vi "Send Connection List.vi"(8 "error in (no error)":errorcluster, 10 "ConnHandlers":refnum<class "Message Enqueuer.lvclass">[](array[class]), 11 "Connection Handler in":refnum<class "Connection Handler.lvclass">) -> (0 "error out":errorcluster, 3 "Connection Handler out":refnum<class "Connection Handler.lvclass">)   [LabVIEW 2017, in "Send Connection List Msg.lvclass"]
uses:
  Connection Handler Messages/Send Connection List Msg/Send Connection List Msg.lvclass
  <vilib>/ActorFramework/Actor/Actor.lvclass
  Connection Handler.lvclass
  Volumes/Data/Users/benji667/Git/BuildFarm/src/LabVIEW/vi.lib/BenjaminR/Build Farm/Actors/Framework/Actor wHelper/Actor wHelper.lvclass
  Volumes/Data/Users/benji667/Git/BuildFarm/src/LabVIEW/vi.lib/BenjaminR/Build Farm/Actors/Framework/Actor wLauncher/Actor wLauncher.lvclass
  Volumes/Data/Users/benji667/Git/BuildFarm/src/LabVIEW/vi.lib/BenjaminR/Build Farm/Actors/Framework/Actor wUI/Actor wUI.lvclass
  Applications/National Instruments/LabVIEW 2017 64-bit/vi.lib/ActorFramework/Actor/Actor.lvclass
  <vilib>/ActorFramework/Message Enqueuer/Message Enqueuer.lvclass
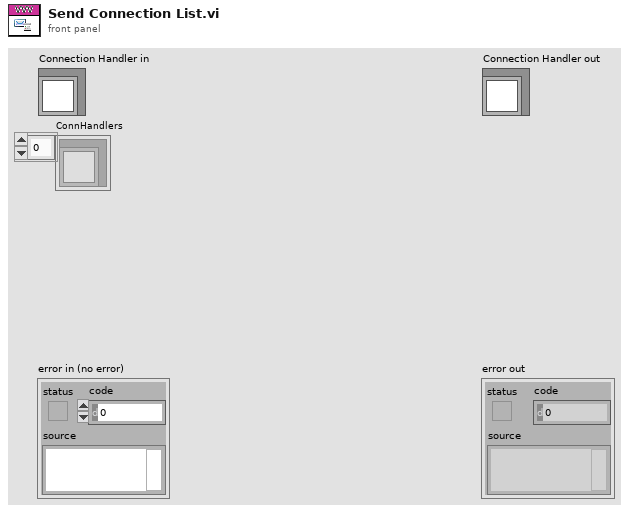
[diagram p1: front panel]
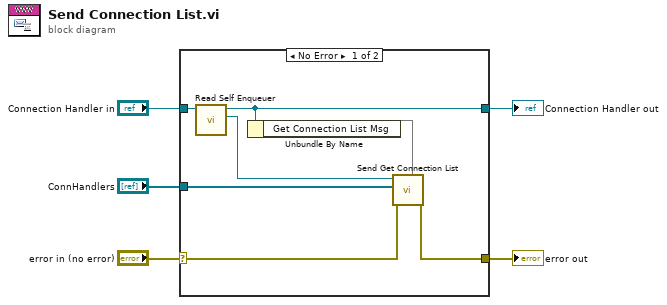
[diagram p0: block diagram]
diagram:
  n1 = case shown="No Error" "error in (no error)" {
    selector: "error in (no error)" -> [w7 w13]
    tunnel: [w6 w13] -> w4
    tunnel: [w10 w12] -> w2
    tunnel: "Connection Handler in" -> [w10 w12]
    tunnel: "ConnHandlers" -> [w8 _]
    frame No Error {
      n2 = call <vilib>:"Read Self Enqueuer.vi"("Actor"=w10) -> ("Self Enqueuer"=w11:refnum<class "Message Enqueuer.lvclass">)  [unwired: 10 in]
      n3 = Unbundle By Name(w10) -> ("Get Connection List Msg"=w9)
      n4 = call "Send Get Connection List.vi"("Message Type"=w9, "error in (no error)"=w7, "ConnHandlers"=w8, "Message Enqueuer"=w11) -> ("error out"=w6:errorcluster)  [unwired: 6 in, 1 out]
    }
    frame Error {
    }
  }
  "error out" <- w4
  "Connection Handler out" <- w2
